vi "Calculate_StabilisationTime.vi"(3 "New Array":dbl[](array[numeric])) -> (0 "Stabilisation time (sec)":dbl, 2 "Stabilisation time (min)":dbl)   [LabVIEW 2018]
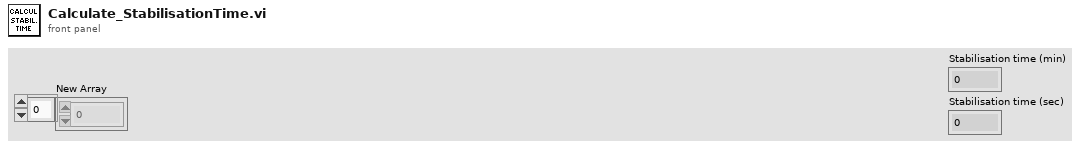
[diagram p1: front panel]
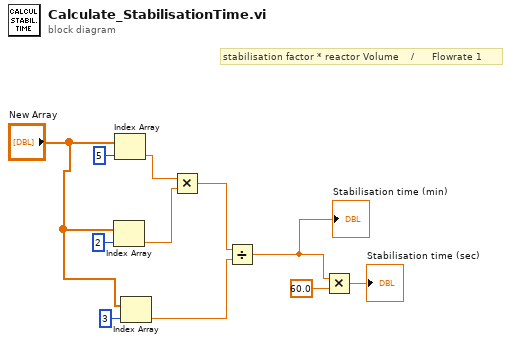
[diagram p0: block diagram]
diagram:
  # "stabilisation factor * reactor Volume    /      Flowrate 1"
  n1 = Index Array(array="New Array", index=2) -> (element=w8:dbl)
  n2 = Index Array(array="New Array", index=5) -> (element=w10:dbl)
  n3 = Index Array(array="New Array", index=3) -> (element=w7:dbl)
  n4 = Multiply(x=w10, y=w8) -> (x*y=w11:dbl)
  n5 = Divide(x=w11, y=w7) -> (x/y=w3:dbl)
  "Stabilisation time (min)" <- w3
  n6 = Multiply(x=w3, y=60.0) -> (x*y=→"Stabilisation time (sec)":dbl)
